vi "MLSD.vi"(8 "error in (no error)":errorcluster, 10 "RemoteDirectory":string, 11 "FTP in":refnum<class "FTP.lvclass">) -> (0 "error out":errorcluster, 2 "Dir-File Info Array":T1[](array[typedef]), 3 "FTP out":refnum<class "FTP.lvclass">)   [LabVIEW 2013, in "FTP.lvlib" / "FTP.lvclass"]
uses:
  FTP.lvclass
  controls/Dir-File Type.ctl
  controls/Dir-File Info.ctl
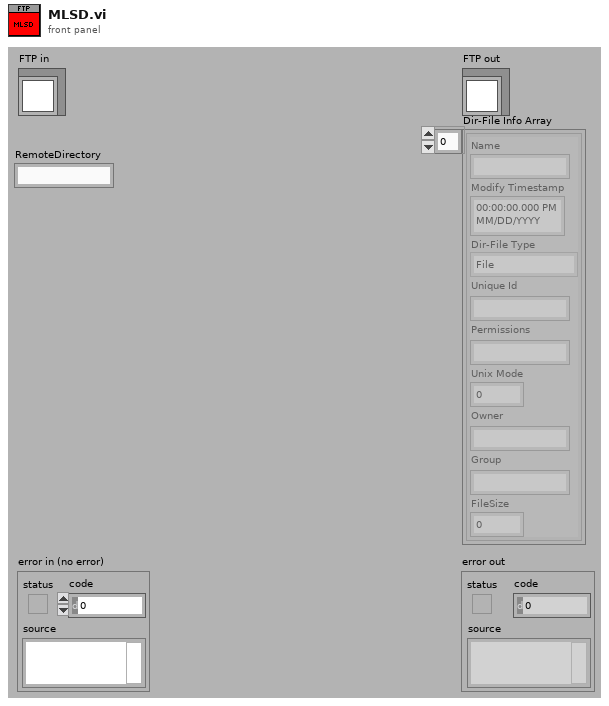
[diagram p1: front panel]
types:
  T1 = typedef "FTP.lvlib/FTP.lvclass/Dir-File Info.ctl" = cluster{"Name":string, "Modify Timestamp":timestamp, "Dir-File Type":T2, "Unique Id":string, "Permissions":string, "Unix Mode":u16, "Owner":string, "Group":string, "FileSize":i64}
  T2 = typedef "FTP.lvlib/FTP.lvclass/Dir-File Type.ctl" = enum16{"File", "Listed Directory", "Parent Directory", "Directory", "Unknown"}
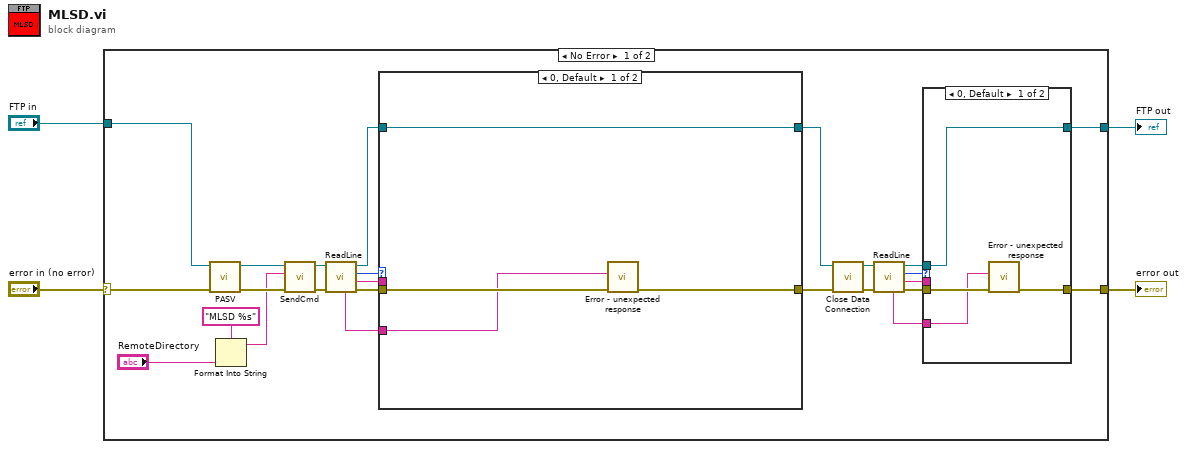
[diagram p0: block diagram]
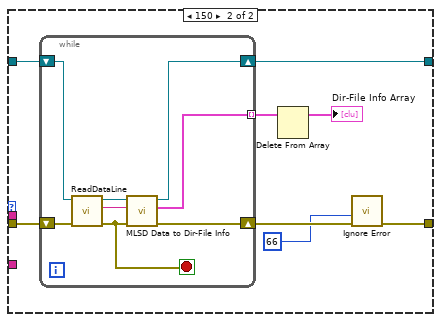
[diagram p3: hidden frame]
diagram:
  n1 = case shown="No Error" "error in (no error)" {
    selector: "error in (no error)" -> [w27 w57]
    tunnel: [w14 w57] -> w3
    tunnel: [w11 w56] -> w1
    tunnel: "FTP in" -> [w26 w56]
    frame No Error {
      n2 = call "PASV.vi"("error in (no error)"=w27, "FTP in"=w26) -> ("error out"=w24:errorcluster, "FTP out"=w25:refnum<class "FTP.lvclass">)  [unwired: 8 in]
      n3 = Format Into String(format string="MLSD %s" ("cmd"), "RemoteDirectory") -> (resulting string=w8:string)  [unwired: 2 in, 1 out]
      n4 = call "SendCmd.vi"("error in (no error)"=w24, "cmd"=w8, "FTP in"=w25) -> ("error out"=w28:errorcluster, "FTP out"=w29:refnum<class "FTP.lvclass">)  [unwired: 7 in]
      n5 = call "ReadLine.vi"("error in (no error)"=w28, "FTP in"=w29) -> ("error out"=w23:errorcluster, "Line"=w21:string, "code"=w22:i32, "FTP out"=w20:refnum<class "FTP.lvclass">, "Full Line"=w5:string)  [unwired: 5 in]
      n6 = case shown="0, Default" w22 {
        tunnel: w23 -> [w38 w47]
        tunnel: w20 -> [w39 w46]
        tunnel: [w37 w42] -> w19
        tunnel: [w39 w45] -> w18
        tunnel: w21 -> [_ _]
        tunnel: w5 -> [w36 _]
        frame 0, Default {
          n7 = call "Error - unexpected response.vi"("error in (no error)"=w38, "Full Response"=w36) -> ("error out"=w37:errorcluster)  [unwired: 9 in]
        }
        frame 150 {
          n8 = while {
            shift-right: [w51] -> w43
            shift-left: w47 -> [w55]
            shift-right: [w50] -> w45
            shift-left: w46 -> [w54]
            tunnel: [w49] -> w44 mode=indexing
            stop <- w48 stop-if-true
            n9 = call "ReadDataLine.vi"("error in (no error)"=w55, "FTP in"=w54) -> ("error out"=w48:errorcluster, "Data"=w53:string, "FTP out"=w52:refnum<class "FTP.lvclass">)  [unwired: 7 in]
            n10 = call "MLSD Data to Dir-File Info.vi"("error in (no error)"=w48, "Data"=w53, "FTP in"=w52) -> ("error out"=w51:errorcluster, "Dir-File Info"=w49:T1, "FTP out"=w50:refnum<class "FTP.lvclass">)  [unwired: 6 in]
          }
          n11 = Delete From Array(array=w44) -> (array with subset deleted=→"Dir-File Info Array":T1[])  [unwired: 2 in, 1 out]
          n12 = call "Ignore Error.vi"("error in"=w43, "code"=66) -> ("error out"=w42:errorcluster)  [unwired: 9 in]
        }
      }
      n13 = call "Close Data Connection.vi"("error in (no error)"=w19, "FTP in"=w18) -> ("error out"=w17:errorcluster, "FTP out"=w16:refnum<class "FTP.lvclass">)  [unwired: 8 in]
      n14 = call "ReadLine.vi"("error in (no error)"=w17, "FTP in"=w16) -> ("error out"=w15:errorcluster, "Line"=w10:string, "code"=w13:i32, "FTP out"=w12:refnum<class "FTP.lvclass">, "Full Line"=w6:string)  [unwired: 5 in]
      n15 = case shown="0, Default" w13 {
        tunnel: w15 -> [w32 w34]
        tunnel: [w31 w34] -> w14
        tunnel: w12 -> [w33 w35]
        tunnel: [w33 w35] -> w11
        tunnel: w10 -> [_ _]
        tunnel: w6 -> [w30 _]
        frame 0, Default {
          n16 = call "Error - unexpected response.vi"("error in (no error)"=w32, "Full Response"=w30) -> ("error out"=w31:errorcluster)  [unwired: 9 in]
        }
        frame 226 {
        }
      }
    }
    frame Error {
    }
  }
  "error out" <- w3
  "FTP out" <- w1
